vi "testCheckQueueFromDdsFull.vi"(8 "error in (no error)":errorcluster) -> (0 "error out":errorcluster)   [LabVIEW 2018]
doc: "Test the checkQueueFull.vi with queueFromDds option."
uses:
  src/TcpServer/TcpServer.lvclass
  src/TcpServerTel/typedef/enqueueOptionsTypeDef.ctl
  src/TcpServer/TcpServer.lvclass/TcpServer.ctl
  src/TcpServerTel/TcpServerTel.lvclass/TcpServerTel.ctl
  src/TcpServerBase/TcpServerBase.lvclass/TcpServerBase.ctl
  src/TcpServerTel/TcpServerTel.lvclass
  home/pcortes/github/ts_labview_tcp_json/src/TcpServerBase/TcpServerBase.lvclass
  <vilib>/addons/_JKI Toolkits/Caraya/classes/Assert/Assert False.vi
  <vilib>/addons/_JKI Toolkits/Caraya/classes/Assert/Assert True.vi
  <vilib>/addons/_JKI Toolkits/Caraya/classes/Test/Test.lvclass
  <vilib>/addons/_JKI Toolkits/Caraya/classes/Assert/Assert.lvclass
  src/TcpServerBase/TcpServerBase.lvclass
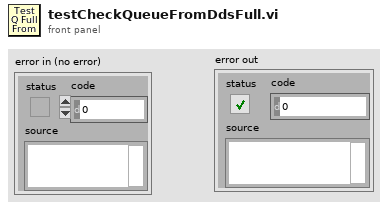
[diagram p1: front panel]
types:
  T1 = typedef "TcpServerTel.lvclass/enqueueOptionsTypeDef.ctl" = enum16{"lossy enqueue", "normal enqueue"}
  T2 = cluster{"cmdServerPort":u16, "telServerPort":u16, "serverTimeout (ms)":i32, "serverBytesToRead":i32, "maxSizeQueueTel":i32, "EnqueueOptions":T1, "timeoutQueueTel (ms)":i32, "tcpClientQueueMaxSize":i32, "timeoutOcc":i32, "timeoutStatusNotifier":i32}
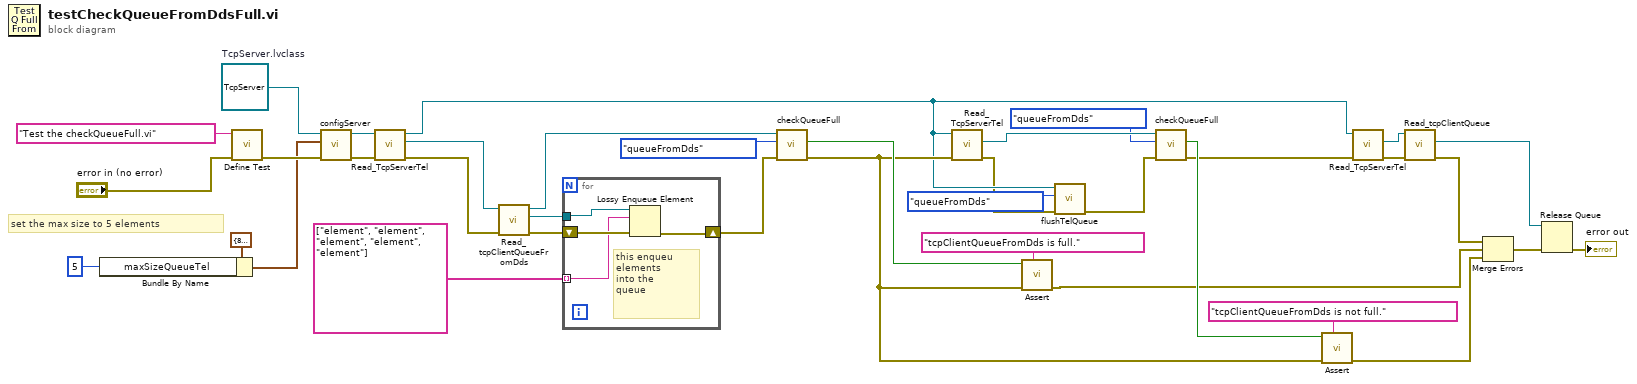
[diagram p0: block diagram]
diagram:
  w26 = refnum<class "TcpServer.lvclass"> refnum  # TcpServer.lvclass
  # "set the max size to 5 elements"
  n1 = Bundle By Name(cluster=T2 {"cmdServerPort"=8888, "telServerPort"=8889, "serverTimeout (ms)"=100, "serverBytesToRead"=32768, "maxSizeQueueTel"=1000, "EnqueueOptions"=enum."lossy enqueue", "timeoutQueueTel (ms)"=50, "tcpClientQueueMaxSize"=1000, "timeoutOcc"=100, "timeoutStatusNotifier"=100} ("ServerConfiguration"), "maxSizeQueueTel"=5 ("telQueueServerMaxSize")) -> (w1:T2)
  n2 = call <vilib>:"Define Test.vi"("error in (no error)"="error in (no error)", "Label (VI Title)"="Test the checkQueueFull.vi") -> ("error out"=w25:errorcluster)  [unwired: 9 in]
  n3 = call "configServer.vi"("error in (no error)"=w25, "ServerConfiguration"=w1, "tcpServer in"=w26) -> ("error out"=w23:errorcluster, "tcpServer out"=w24:refnum<class "TcpServer.lvclass">)  [unwired: 7 in]
  n4 = call "Read_TcpServerTel.vi"("error in (no error)"=w23, "TcpServer in"=w24) -> ("error out"=w11:errorcluster, "TcpServerTel.lvclass"=w9:refnum<class "TcpServerTel.lvclass">, "TcpServer out"=w6:refnum<class "TcpServer.lvclass">)  [unwired: 7 in]
  n5 = call "Read_tcpClientQueueFromDds.vi"("error in (no error)"=w11, "TcpServerTel in"=w9) -> ("error out"=w10:errorcluster, "tcpClientQueueFromDds"=w8:refnum<queue>, "TcpServerTel out"=w7:refnum<class "TcpServerTel.lvclass">)  [unwired: 7 in]
  n6 = for {
    shift-right: [w40] -> w22
    shift-left: w10 -> [w41]
    tunnel: string[] ["element", "element", "element", "element", "element"] -> [w38] mode=indexing
    tunnel: w8 -> [w39]
    # "this enqueu\nelements\ninto the\nqueue"
    n7 = Lossy Enqueue Element(queue=w39, element=w38, error in (no error)=w41) -> (error out=w40:errorcluster)  [unwired: 3 out]
  }
  n8 = call "checkQueueFull.vi"("error in (no error)"=w22, "queueName"=enum16{"queueFromDds", "queueToDds"}."queueFromDds", "tcpServerTel in"=w7) -> ("error out"=w20:errorcluster, "queueFull"=w32:bool)  [unwired: 6 in, 1 out]
  n9 = call "Read_TcpServerTel.vi"("error in (no error)"=w20, "TcpServer in"=w6) -> ("error out"=w5:errorcluster, "TcpServerTel.lvclass"=w14:refnum<class "TcpServerTel.lvclass">)  [unwired: 7 in, 1 out]
  n10 = call-poly <vilib>:"Assert.vi"("Label"="tcpClientQueueFromDds is full.", "error in (no error)"=w20, "True?"=w32) -> ("error out"=w17:errorcluster)  [unwired: 8 in]
  n11 = call "flushTelQueue.vi"("error in (no error)"=w5, "queueName"=enum16{"queueFromDds", "queueToDds"}."queueFromDds", "TcpServer in"=w6) -> ("error out"=w4:errorcluster)  [unwired: 6 in, 2 out]
  n12 = call "checkQueueFull.vi"("error in (no error)"=w4, "queueName"=enum16{"queueFromDds", "queueToDds"}."queueFromDds", "tcpServerTel in"=w14) -> ("error out"=w18:errorcluster, "queueFull"=w19:bool)  [unwired: 6 in, 1 out]
  n13 = call-poly <vilib>:"Assert.vi"("Label"="tcpClientQueueFromDds is not full.", "error in (no error)"=w20, "False?"=w19) -> ("error out"=w16:errorcluster)  [unwired: 8 in]
  n14 = call "Read_TcpServerTel.vi"("error in (no error)"=w18, "TcpServer in"=w6) -> ("error out"=w31:errorcluster, "TcpServerTel.lvclass"=w30:refnum<class "TcpServerTel.lvclass">)  [unwired: 7 in, 1 out]
  n15 = call "Read_tcpClientQueue.vi"("error in (no error)"=w31, "TcpServerBase in"=w30) -> ("error out"=w28:errorcluster, "tcpClientQueue"=w29:refnum<queue>)  [unwired: 7 in, 1 out]
  n16 = Merge Errors(w28, w17, w16) -> (w33:errorcluster)
  n17 = Release Queue(queue=w29, error in (no error)=w33) -> (error out=→"error out":errorcluster)  [unwired: 1 in, 2 out]
